vi "TCP Multiple Connections - Server.vi"() -> ()   [LabVIEW 2023]
doc: "This is the TCP server VI that supports multiple connections from client VIs."
uses:
  controls/TCP Multiple Connections State.ctl
  controls/TCP Multiple Connections Data.ctl
panel:
  out "WfS":dbl
  out "A1_ITT":dbl
  out "A1_NSA":dbl
  in  "WfS":dbl(slide) scale=0.0..10000.0
  in  "A1_ITT":dbl(slide) scale=0.0..1000.0
  in  "A1_NSA":dbl(slide) scale=0.0..100.0
  in  "N2I":dbl(slide) scale=0.0..10000.0
  in  "N1I":dbl(slide) scale=0.0..10000.0
  out "Read Data String":string
  out "Sent String":string
  out "N2I":dbl
  in  "Stop":bool
  out "N1I":dbl
  out "# of Connections":i32
  # "CERES Simulator Controller Station\n\n1. Run the VI.\n2. Run Pilot on delta1."
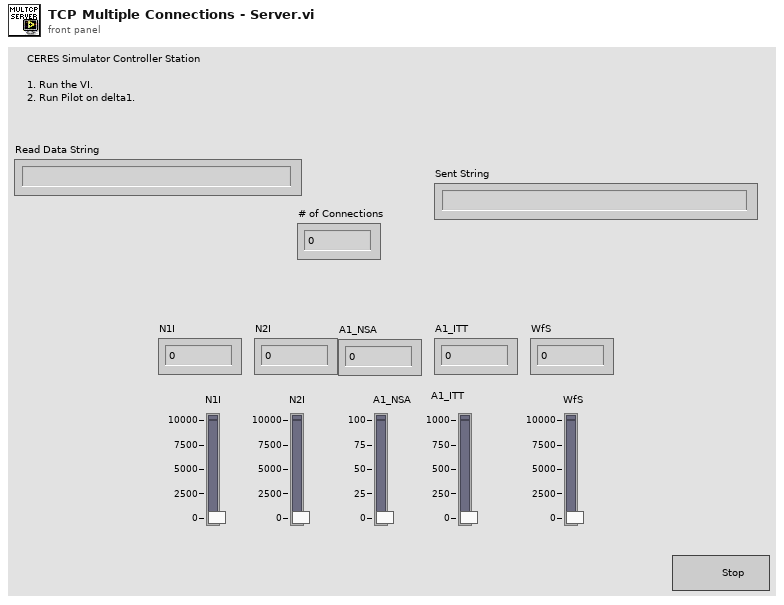
[diagram p1: front panel]
types:
  T1 = typedef "TCP Multiple Connections Data.ctl" = cluster{"Clients":refnum<k5>[], "Listener":refnum<k5>}
  T2 = typedef "TCP Multiple Connections State.ctl" = enum16{"Initialize", "Status Check", "Send Data", "Stop"}
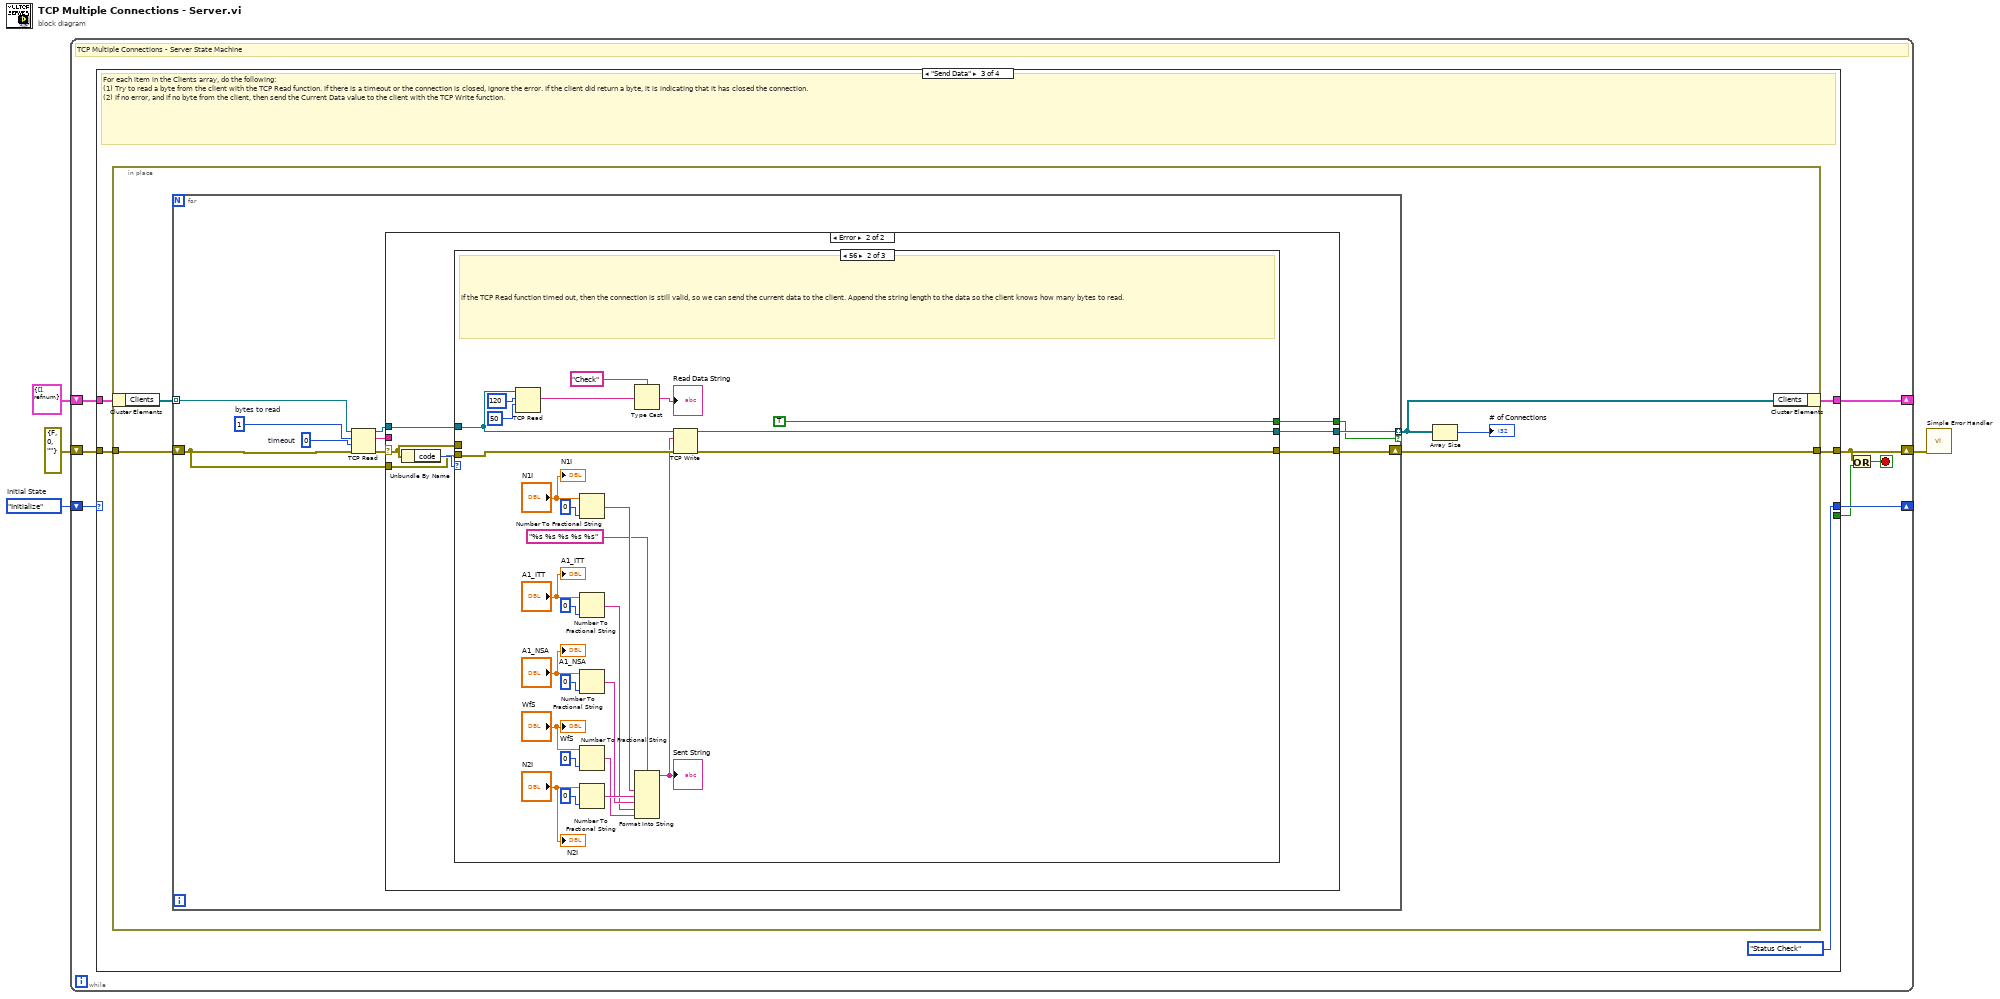
[diagram p0: block diagram]
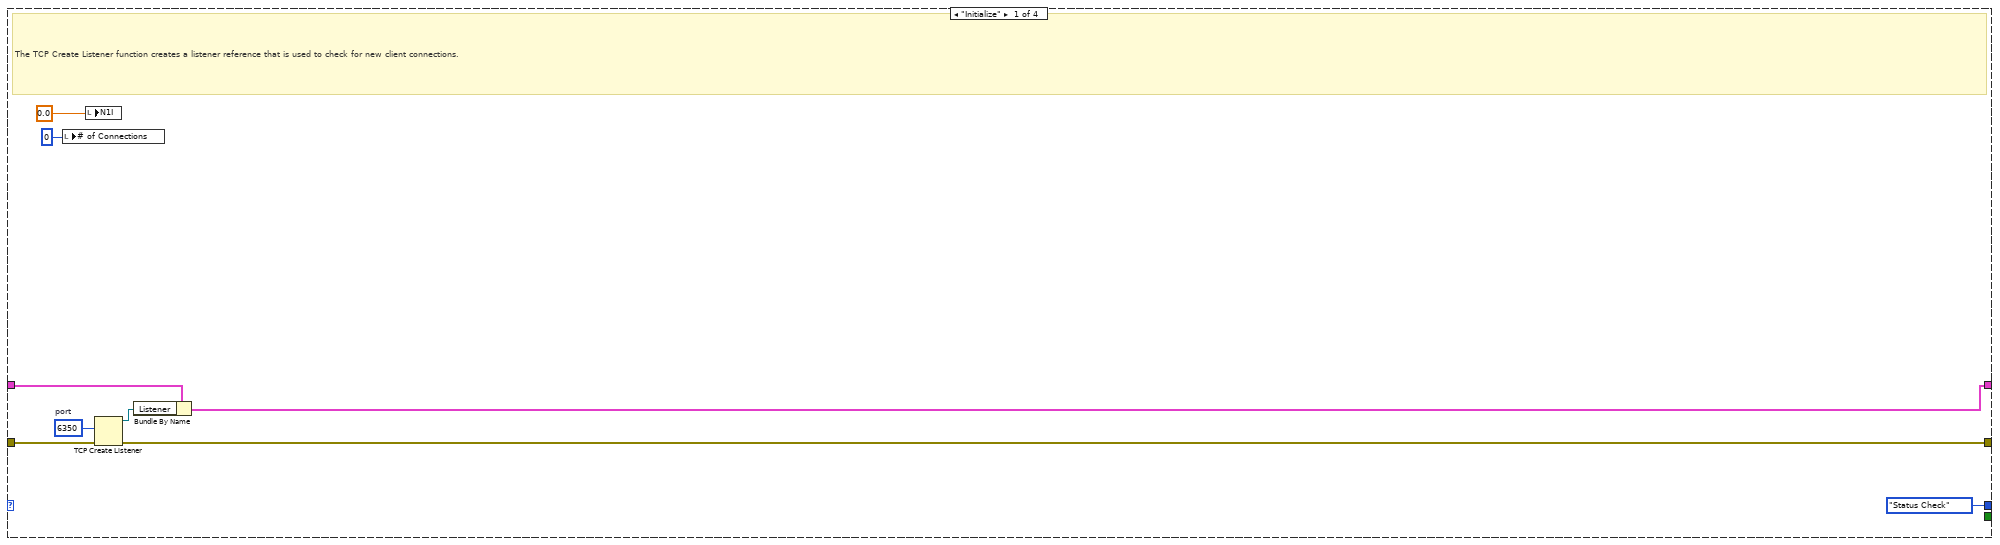
[diagram p2: hidden frame]
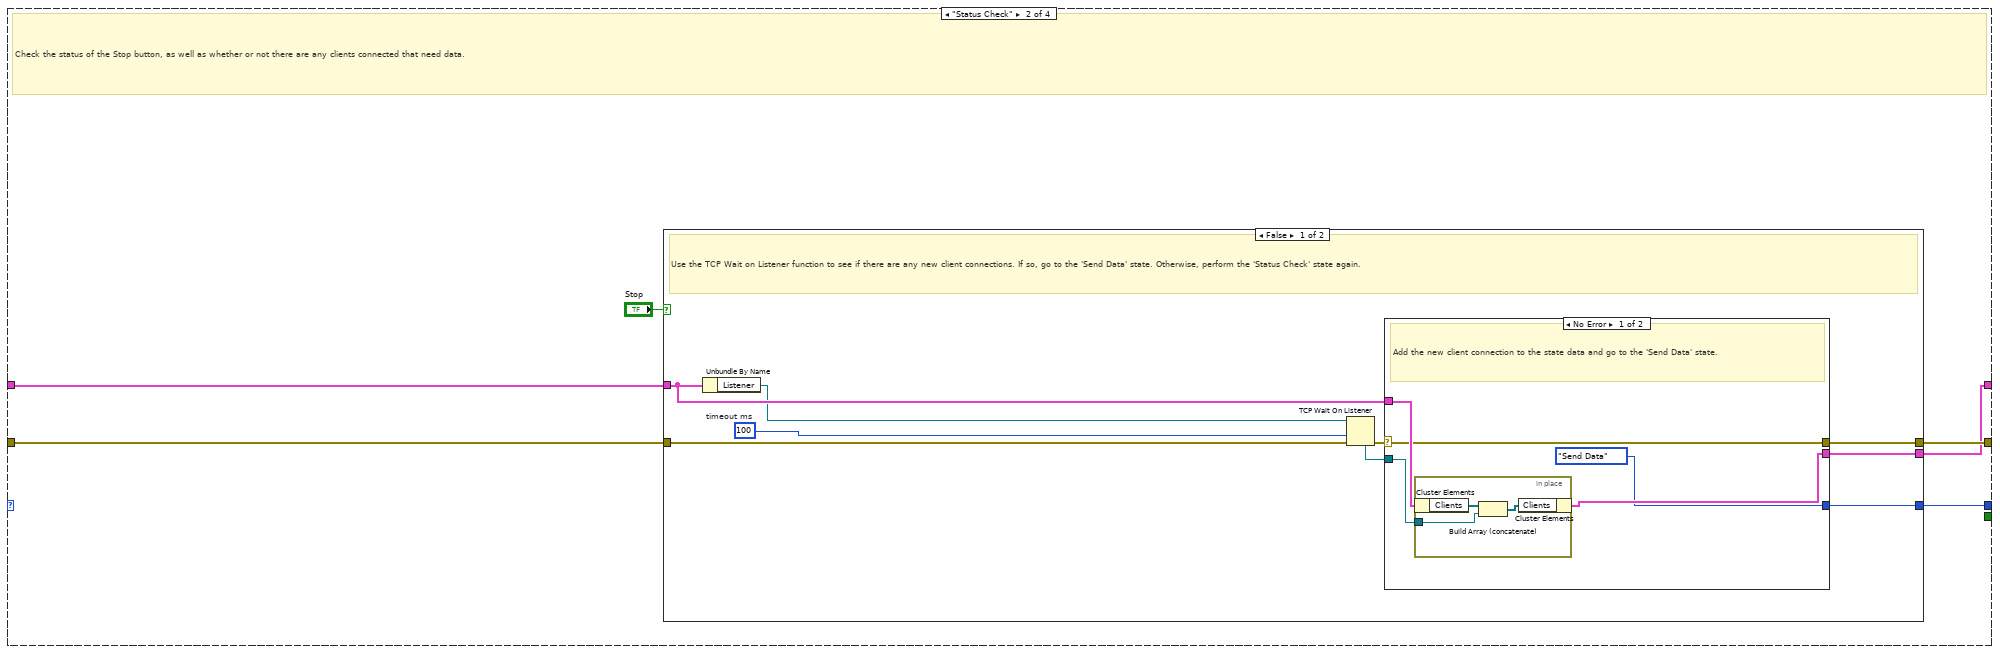
[diagram p3: hidden frame]
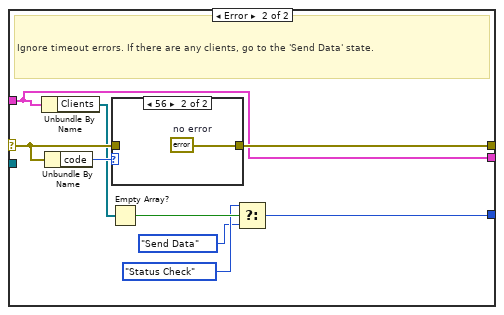
[diagram p4: hidden frame]
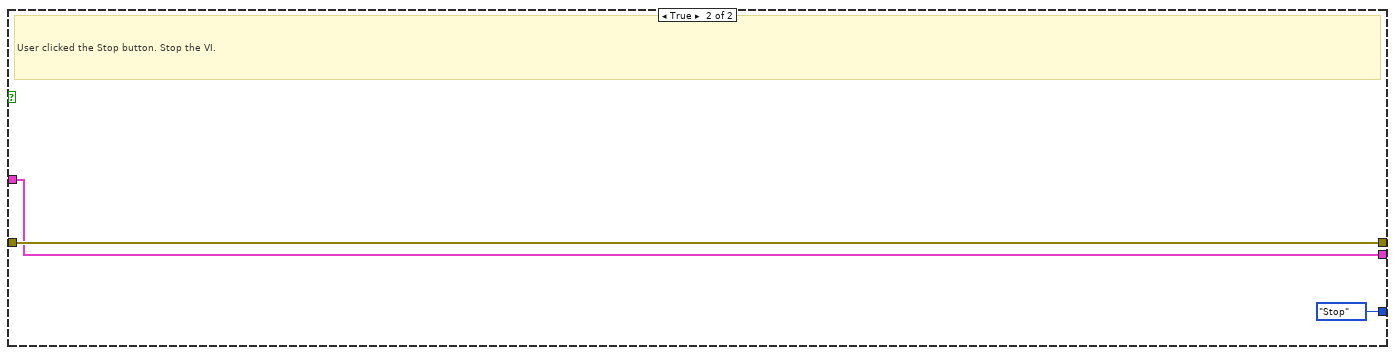
[diagram p6: hidden frame]
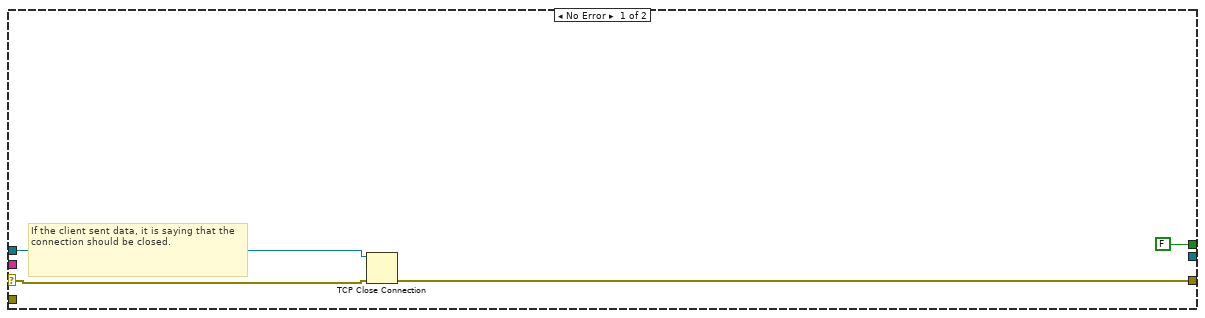
[diagram p7: hidden frame]
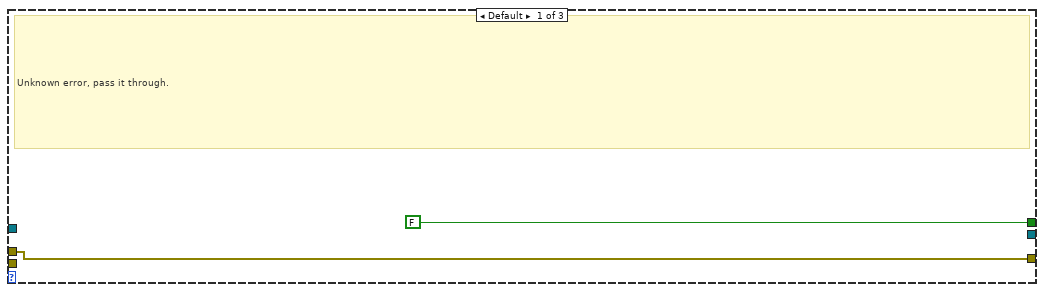
[diagram p8: hidden frame]
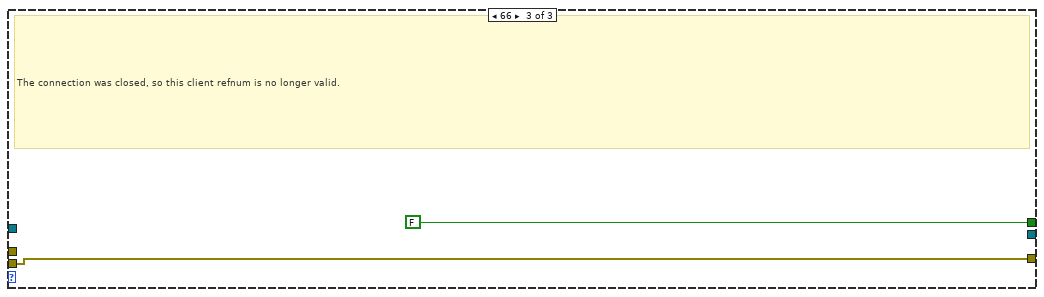
[diagram p9: hidden frame]
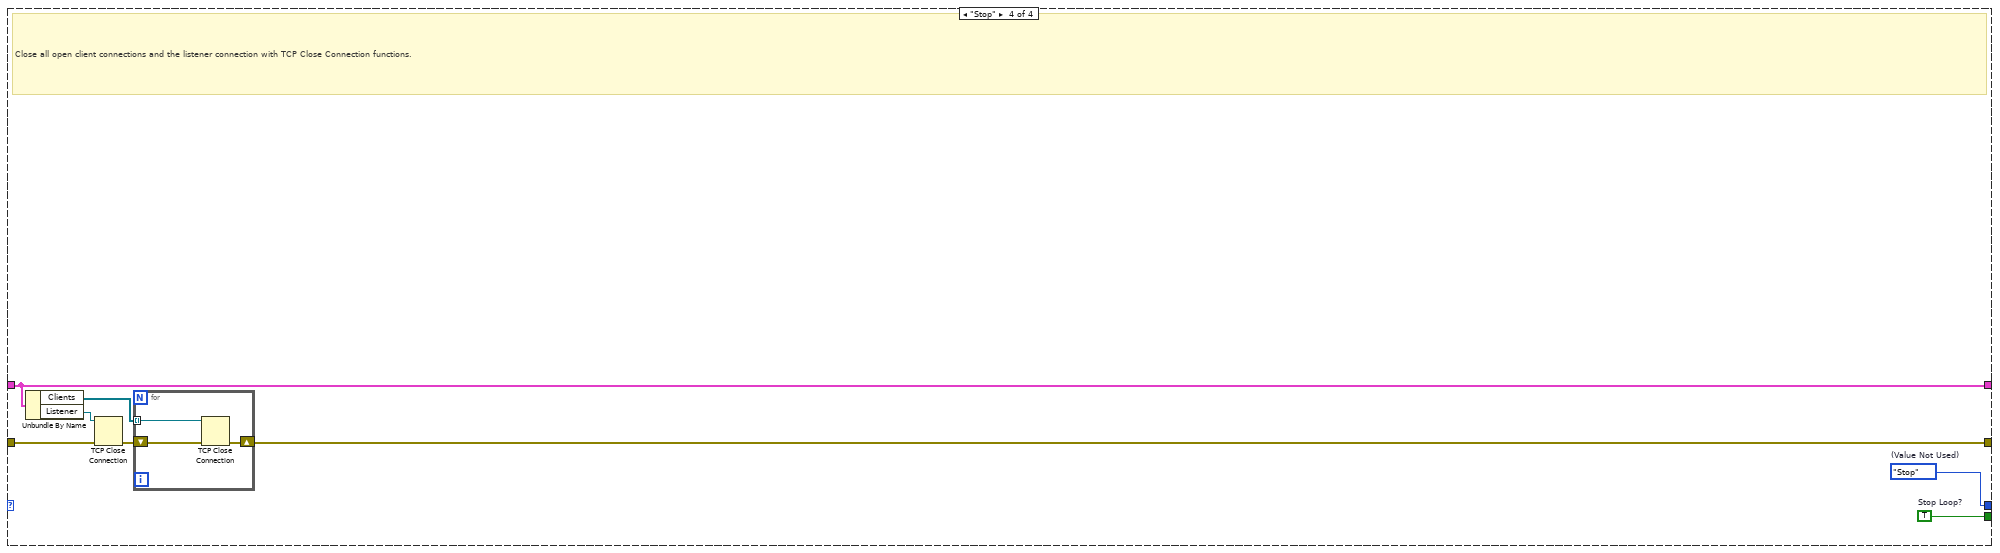
[diagram p10: hidden frame]
diagram:
  w4 = TCP_Multiple_Connections_State."Initialize"  # Initial State
  n1 = while {
    shift-right: [w11] -> _
    shift-left: w4 -> [w12]
    shift-right: [w9] -> _
    shift-left: T1 {"Clients"=[], "Listener"=refnum} ("Data") -> [w10]
    shift-right: [w5] -> w1
    shift-left: errorcluster {"status"=FALSE, "code"=0, "source"=""} ("error constant") -> [w8]
    stop <- w6 stop-if-true
    # "TCP Multiple Connections - Server State Machine"
    n2 = case shown="\"Send Data\"" w12 {
      tunnel: [TCP_Multiple_Connections_State."Status Check" ("States") w27 TCP_Multiple_Connections_State."Status Check" ("States") w121] -> w11
      tunnel: [_ _ _ w128] -> w7
      tunnel: w10 -> [w19 w23 w61 w127]
      tunnel: [w18 w22 w60 w127] -> w9
      tunnel: w8 -> [w21 w26 w63 w126]
      tunnel: [w20 w25 w62 w124] -> w5
      frame "Initialize" {
        w16 = u16 6350  # port
        # "The TCP Create Listener function creates a listener reference that is used to check for new client connections."
        n3 = local write "# of Connections"(0 ("Number of Client Connections")) -> ()
        n4 = local write "N1I"(0.0 ("Current Data")) -> ()
        n5 = TCP Create Listener(8:w21, 10:w16) -> (0:w20:errorcluster, 3:w17:refnum<k5>)  [unwired: 4 out]
        n6 = Bundle By Name(cluster=w19, "Listener"=w17) -> (w18:T1)
      }
      frame "Status Check" {
        # "Check the status of the Stop button, as well as whether or not there are any clients connected that need data."
        n7 = case shown="False" "Stop" {
          tunnel: [w36 TCP_Multiple_Connections_State."Stop" ("States")] -> w27
          tunnel: w26 -> [w35 w58]
          tunnel: [w28 w58] -> w25
          tunnel: w23 -> [w31 w57]
          tunnel: [w30 w57] -> w22
          frame False {
            w34 = 100  # timeout ms
            # "Use the TCP Wait on Listener function to see if there are any new client connections. If so, go to the 'Send Data' state. Otherwise, perform the 'Status Check' state again."
            n8 = Unbundle By Name(w31) -> ("Listener"=w29:refnum<k5>)
            n9 = TCP Wait On Listener(8:w35, 9:w34, 11:w29) -> (0:w33:errorcluster, 4:w32:refnum<k5>)  [unwired: 4 out]
            n10 = case shown="No Error" w33 {
              selector: w33 -> [w39 w53]
              tunnel: [TCP_Multiple_Connections_State."Send Data" ("States") w47] -> w36
              tunnel: w32 -> [w40 _]
              tunnel: w31 -> [w41 w50]
              tunnel: [w38 w50] -> w30
              tunnel: [w39 w51] -> w28
              frame No Error {
                # "Add the new client connection to the state data and go to the 'Send Data' state."
                n11 = in-place {
                  in-place-border: w40 -> [w42]
                  n12 = in-place-cluster #1(w41) -> ("Clients"=w44:refnum<k5>[])
                  n13 = Build Array (concatenate)(w44, w42) -> (w43:refnum<k5>[])
                  n14 = in-place-cluster #1("Clients"=w43) -> (w38:T1)
                }
              }
              frame Error {
                # "Ignore timeout errors. If there are any clients, go to the 'Send Data' state."
                n15 = Unbundle By Name(w50) -> ("Clients"=w49:refnum<k5>[])
                n16 = Unbundle By Name(w53) -> ("code"=w52:i32)
                n17 = Empty Array?(array=w49) -> (empty?=w48:bool)
                n18 = case shown="56" w52 {
                  tunnel: w53 -> [w54 _]
                  tunnel: [w54 w55] -> w51
                  frame Default {
                  }
                  frame 56 {
                    w55 = errorcluster {"status"=FALSE, "code"=0, "source"=""}  # no error
                  }
                }
                n19 = Select(t=TCP_Multiple_Connections_State."Status Check" ("States"), s=w48, f=TCP_Multiple_Connections_State."Send Data" ("States")) -> (s? t:f=w47:T2)
              }
            }
          }
          frame True {
            # "User clicked the Stop button. Stop the VI."
          }
        }
      }
      frame "Send Data" {
        # "For each item in the Clients array, do the following:\n(1) Try to read a byte from the client with the TCP Read function. If there is a timeout or the connection is closed, ignore the error. If the client did return a byte, it is indicating that it has closed the connection.\n(2) If no error, and if no byte from the client, then send the Current Data value to the client with the TCP Write function."
        n20 = in-place {
          in-place-border: w63 -> [w68]
          in-place-border: [w67] -> w62
          n21 = in-place-cluster #2(w61) -> ("Clients"=w65:refnum<k5>[])
          n22 = for {
            tunnel: w65 -> [w78] mode=indexing
            shift-right: [w71] -> w67
            shift-left: w68 -> [w70]
            tunnel: [w73] -> w64 mode=indexing if=w72
            w76 = 0  # timeout
            w69 = 1  # bytes to read
            n23 = TCP Read(connection ID=w78, bytes to read=w69, error in (no error)=w70, 9:w76) -> (connection ID out=w77:refnum<k5>, data out=w74:string, error out=w75:errorcluster)  [unwired: 1 out]
            n24 = case shown="Error" w75 {
              selector: w75 -> [w81 w88]
              tunnel: w77 -> [w82 w85]
              tunnel: w74 -> [_ _]
              tunnel: [_ w83] -> w73
              tunnel: [FALSE w84] -> w72
              tunnel: [w79 w87] -> w71
              tunnel: w70 -> [_ w86]
              frame No Error {
                # "If the client sent data, it is saying that the connection should be closed."
                # "If the client sent data, it is saying that the connection should be closed."
                n25 = TCP Close Connection(connection ID=w82, error in (no error)=w81) -> (error out=w79:errorcluster)  [unwired: 2 out]
              }
              frame Error {
                # "Ignore connection closed and timeout errors"
                n26 = Unbundle By Name(w88) -> ("code"=w89:i32)
                n27 = case shown="56" w89 {
                  tunnel: w88 -> [w91 _ _]
                  tunnel: [w91 w118 w120] -> w87
                  tunnel: w86 -> [_ w115 w120]
                  tunnel: w85 -> [_ w108 _]
                  tunnel: [FALSE TRUE FALSE] -> w84
                  tunnel: [_ w117 _] -> w83
                  frame Default {
                    # "Unknown error, pass it through."
                  }
                  frame 56 {
                    # "If the TCP Read function timed out, then the connection is still valid, so we can send the current data to the client. Append the string length to the data so the client knows how many bytes to read."
                    n28 = TCP Read(connection ID=w108, bytes to read=120, 9:50) -> (data out=w106:string)  [unwired: 1 in, 3 out]
                    n29 = Number To Fractional String(number="N1I", precision (6)=0) -> (F-format string=w112:string)  [unwired: 2 in]
                    n30 = Number To Fractional String(number="A1_ITT", precision (6)=0) -> (F-format string=w96:string)  [unwired: 2 in]
                    n31 = Number To Fractional String(number="A1_NSA", precision (6)=0) -> (F-format string=w97:string)  [unwired: 2 in]
                    n32 = Number To Fractional String(number="WfS", precision (6)=0) -> (F-format string=w95:string)  [unwired: 2 in]
                    n33 = Number To Fractional String(number="N2I", precision (6)=0) -> (F-format string=w110:string)  [unwired: 2 in]
                    n34 = Type Cast(type="Check", x=w106) -> (*(type *) &x=→"Read Data String":string)
                    n35 = Format Into String(format string="%s %s %s %s %s", w112, w110, w97, w96, w95) -> (resulting string=w109:string)  [unwired: 2 in, 1 out]
                    "Sent String" <- w109
                    n36 = TCP Write(connection ID=w108, data in=w109, error in (no error)=w115) -> (connection ID out=w117:refnum<k5>, error out=w118:errorcluster)  [unwired: 2 out]
                    "N1I" <- "N1I"
                    "N2I" <- "N2I"
                    "A1_NSA" <- "A1_NSA"
                    "A1_ITT" <- "A1_ITT"
                    "WfS" <- "WfS"
                  }
                  frame 66 {
                    # "The connection was closed, so this client refnum is no longer valid."
                  }
                }
              }
            }
          }
          n37 = Array Size(array=w64) -> (size(s)=→"# of Connections":i32)
          n38 = in-place-cluster #2("Clients"=w64) -> (w60:T1)
        }
      }
      frame "Stop" {
        w121 = TCP_Multiple_Connections_State."Stop"  # (Value Not Used)
        w128 = TRUE  # Stop Loop?
        # "Close all open client connections and the listener connection with TCP Close Connection functions."
        n39 = Unbundle By Name(w127) -> ("Clients"=w125:refnum<k5>[], "Listener"=w122:refnum<k5>)
        n40 = TCP Close Connection(connection ID=w122, error in (no error)=w126) -> (error out=w123:errorcluster)  [unwired: 1 in, 1 out]
        n41 = for {
          shift-right: [w130] -> w124
          shift-left: w123 -> [w131]
          tunnel: w125 -> [w129] mode=indexing
          n42 = TCP Close Connection(connection ID=w129, error in (no error)=w131) -> (error out=w130:errorcluster)  [unwired: 1 in, 1 out]
        }
      }
    }
    n43 = Or(x=w5, y=w7) -> (x .or. y?=w6:bool)
  }
  n44 = call <vilib>:"Simple Error Handler.vi"("error in (no error)"=w1) -> ()  [unwired: 4 in, 5 out]
